vi "Simple DMM SCAN DER - Loop.vi"() -> ()   [LabVIEW 2021]
uses:
  DMM SCAN DER/Typedefs/Scan configuration.ctl
  <instrlib>/niDMM/nidmm.llb/niDMM Resolution in Digits.ctl
  DMM SCAN DER/Typedefs/Formatted measurement.ctl
  DMM SCAN DER/Typedefs/Scan Resource Names.ctl
  DMM SCAN DER/DMM_Scan DAQ Ext RLY.lvlib
panel:
  in  "stop":bool
  out "Total Scan Time (s)":dbl=0.4806106999999429 format="%#.3p"
  out "Formatted Measurements":T1[](array[typedef])=[{"Channel"="ch0", "Switch Time"=0.07685059999994337, "Formatted Measurement"="9.89411V (dc)", "Out of Range"=FALSE}, {"Channel"="ch1", "Switch Time"=0.07492750000028536, "Formatted Measurement"="96.2760mV (dc)", "Out of Range"=FALSE}, {"Channel"="ch2", "Switch Time"=0.3288286999995762, "Formatted Measurement"="9.377907uA (dc)", "Out of Range"=FALSE}] {"Switch Time" format="%#_3p"}
  in  "Scan Configuration":T2[](array[typedef])=[{"Channel"="ch0", "Resolution in Digits"=5.5, "Range and Function"=enum."DC 10 V"}, {"Channel"="ch1", "Resolution in Digits"=5.5, "Range and Function"=enum."DC 100 mV"}, {"Channel"="ch2", "Resolution in Digits"=6.5, "Range and Function"=enum."DC 10 uA"}] {"Resolution in Digits" items=["3 1/2"=3.5, "4 1/2"=4.5, "5 1/2"=5.5, "6 1/2"=6.5, "7 1/2"=7.5]}
  out "error out":errorcluster
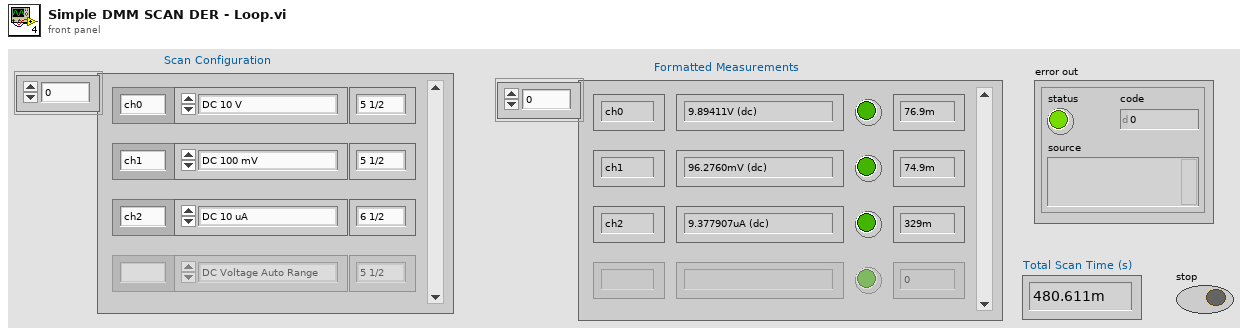
[diagram p1: front panel]
types:
  T1 = typedef "DMM_Scan DAQ Ext RLY.lvlib/Formatted measurement.ctl" = cluster{"Channel":string, "Switch Time":dbl, "Formatted Measurement":string, "Out of Range":bool}
  T2 = typedef "DMM_Scan DAQ Ext RLY.lvlib/Scan configuration.ctl" = cluster{"Channel":string, "Resolution in Digits":T3, "Range and Function":enum16{"DC Voltage Auto Range", "DC 100 mV", "DC 1 V ", "DC 10 V", "DC 100 V", "DC 300 V", " ", "AC Voltage Auto Range", "AC 50 mV", "AC 200 mV", "AC 500 mV", "AC 2 V", "AC 5 V", "AC 20 V", "AC 50 V", "AC 300 V", "  ", "DC Current Auto Range", "DC 1 uA", "DC 10 uA", "DC 100 uA", "DC 1 mA", "DC 10 mA", "DC 20 mA", "DC 100 mA", "DC 200 mA", "DC 1 A", "DC 3 A", "   ", "AC Current Auto Range", "AC 100 uA", "AC 1 mA", "AC 10 mA", "AC 100 mA", "AC 500 mA", "AC 1 A", "AC 3 A", "    ", "Resistance Auto Range", "Res 100 Ohm", "Res 1 kOhm", "Res 10 kOhm", "Res 100 kOhm", "Res 1 MOhm", "Res 10 MOhm", "Res 100 MOhm", "Res 5 GOhm", "     ", "Frequency AC Auto Range", "Freq AC 50 mV", "Freq AC 500 mV", "Freq AC 5 V", "Freq AC 50 V", "Freq AC 300 V", "      ", "Period AC Auto Range", "Period AC 50 mV", "Period AC 500 mV", "Period AC 5 V", "Period AC 50 V", "Period AC 300 V"}}
  T3 = typedef "niDMM Resolution in Digits.ctl" = dbl
  T4 = cluster{"Min Channel Voltage":u32, "Max Channel Voltage":u32, "Min Channel Current":u32, "Max Channel Current":u32, "N Shift Shunt to Min Channel Current":u32}
  T5 = typedef "DMM_Scan DAQ Ext RLY.lvlib/Scan Resource Names.ctl" = cluster{"DMM Resource Name":refnum<k15>, "DAQ Resource Physical Channels Names":tag}
  T6 = typedef "DMM_Scan DAQ Ext RLY.lvlib/Scan Resource Handles Out.ctl" = cluster{"DMM Handle":refnum<k15>, "DAQmx Task Out":refnum<k21>, "Relays Status Array":bool[], "N Shift Shunt":u32, "Close all Shunts?":bool, "Relays Debounce Time (ms)":u32}
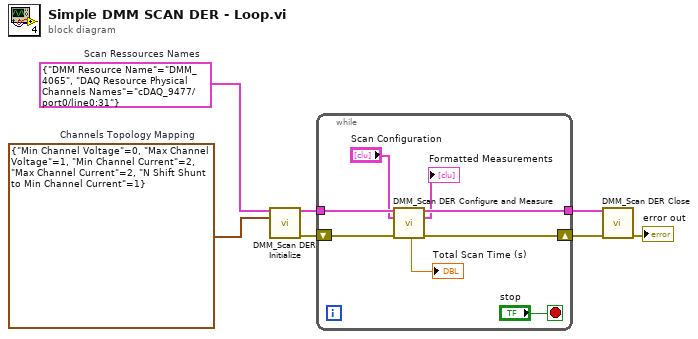
[diagram p0: block diagram]
diagram:
  w1 = T4 {"Min Channel Voltage"=0, "Max Channel Voltage"=1, "Min Channel Current"=2, "Max Channel Current"=2, "N Shift Shunt to Min Channel Current"=1}  # Channels Topology Mapping
  w5 = T5 {"DMM Resource Name"="DMM_4065", "DAQ Resource Physical Channels Names"="cDAQ_9477/port0/line0:31"}  # Scan Ressources Names
  n1 = call "DMM_Scan DER Initialize.vi"("Scan Resources Names"=w5, "Channels Topology Mapping"=w1) -> ("Scan Resources Handles Out"=w4:T6, "error out"=w7:errorcluster)  [unwired: 11 in, 1 out]
  n2 = while {
    tunnel: w4 -> [w13]
    tunnel: [w12] -> w3
    shift-right: [w14] -> w6
    shift-left: w7 -> [w15]
    stop <- "stop" stop-if-true
    n3 = call "DMM_Scan DER Configure and Measure.vi"("Scan Resources Handles In"=w13, "Scan Configuration"="Scan Configuration", "error in"=w15) -> ("Scan Resources Handles Out"=w12:T6, "Formatted Measurements"=→"Formatted Measurements":T1[], "Total Scan Time (s)"=→"Total Scan Time (s)":dbl, "error out"=w14:errorcluster)  [unwired: 7 in, 2 out]
  }
  n4 = call "DMM_Scan DER Close.vi"("Scan Resources Handles In"=w3, "error in"=w6) -> ("error out"=→"error out":errorcluster)  [unwired: 13 in]
